vi "Serial_Communication.vi"() -> ()   [LabVIEW 2013]
uses:
  <vilib>/Instr/_visa.llb/VISA Configure Serial Port (Instr).vi
panel:
  in  "Send Button":bool
  in  "Send Data":string
  in  "Stop":bool
  out "Data Received":string
  in  "COM Port":refnum<visa-resource-name>
  # "Embedded Laboratory"
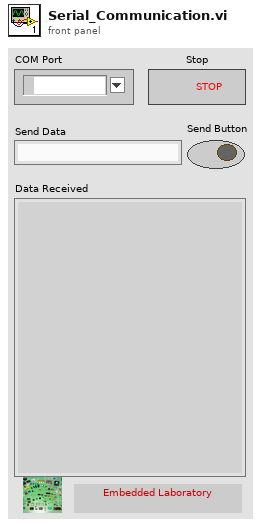
[diagram p1: front panel]
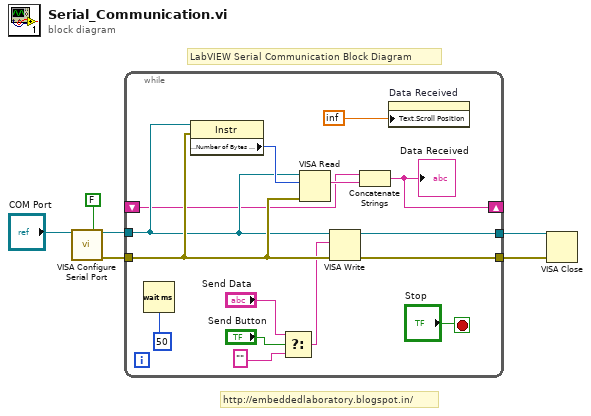
[diagram p0: block diagram]
diagram:
  # "http://embeddedlaboratory.blogspot.in/"
  # "LabVIEW Serial Communication Block Diagram"
  n1 = call-poly "VISA Configure Serial Port"("VISA resource name"="COM Port", "Enable Termination\nChar (T)"=FALSE ("Enable Termination\nChar (T)")) -> ("VISA resource name out"=w4:refnum<visa-resource-name>, "error out"=w1:errorcluster)  [unwired: 12 in]
  n2 = while {
    tunnel: w4 -> [w16]
    tunnel: [w21] -> w3
    tunnel: [w20] -> w2
    tunnel: w1 -> [w17]
    shift-right: [w14] -> _
    shift-left: _ -> [w13]
    stop <- "Stop" stop-if-true
    n3 = Wait (ms)(milliseconds to wait=u32 50) -> ()  [unwired: 1 out]
    n4 = property class="Instr"(reference=w16, error in=w17) -> ("Serial Settings:Number of Bytes at Serial Port"=w18:u32)  [unwired: 2 out]
    n5 = Select(t="Send Data", s="Send Button", f="") -> (s? t:f=w9:string)
    n6 = VISA Read(VISA resource name=w16, byte count=w18, error in (no error)=w17) -> (read buffer=w15:string)  [unwired: 3 out]
    n7 = VISA Write(VISA resource name=w16, write buffer=w9, error in (no error)=w17) -> (VISA resource name out=w21:refnum<visa-resource-name>, error out=w20:errorcluster)  [unwired: 1 out]
    n8 = Concatenate Strings(w13, w15) -> (w14:string)
    "Data Received" <- w14
    n9 = property on="Data Received" class="Str"("Text.Scroll Position"=inf) -> ()  [unwired: 2 in, 2 out]
  }
  n10 = VISA Close(VISA resource name=w3, error in (no error)=w2) -> ()  [unwired: 1 out]
